vi "Save data.vi"(10 "Auto Data":T1(array[cluster]), 11 "File":path) -> ()   [LabVIEW 2012]
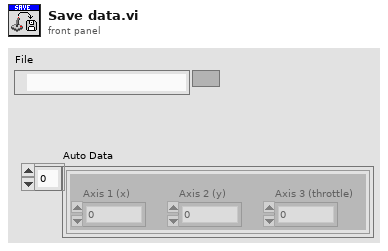
[diagram p1: front panel]
types:
  T1 = cluster{"Axis 1 (x)":dbl, "Axis 2 (y)":dbl, "Axis 3 (throttle)":dbl}[]
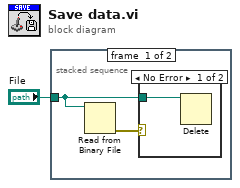
[diagram p0: block diagram]
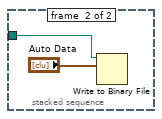
[diagram p3: hidden frame]
diagram:
  n1 = stacked-sequence {
    tunnel: "File" -> [w2 w5]
    frame #0 {
      n2 = Read from Binary File(11:w2) -> (0:w3:errorcluster)  [unwired: 5 in, 3 out]
      n3 = case shown="No Error" w3 {
        tunnel: w2 -> [w4 _]
        frame No Error {
          n4 = Delete(path (use dialog)=w4) -> ()  [unwired: 4 in, 3 out]
        }
        frame Error {
        }
      }
    }
    frame #1 {
      n5 = Write to Binary File(file (use dialog)=w5, data="Auto Data") -> ()  [unwired: 4 in, 3 out]
    }
  }
